vi "Byte Buffer.Clear.vi"(8 "error in (no error)":errorcluster, 11 "Byte Buffer in":refnum<class "Byte Buffer.lvclass">) -> (0 "error out":errorcluster, 3 "Byte Buffer out":refnum<class "Byte Buffer.lvclass">)   [LabVIEW 2016, in "VeriStand Data.lvlib" / "Byte Buffer.lvclass"]
doc: "Sets all bytes in the provided <B>buffer</B> to zero."
uses:
  Byte Buffer.lvclass
  Byte Buffer.lvclass/Byte Buffer.ctl
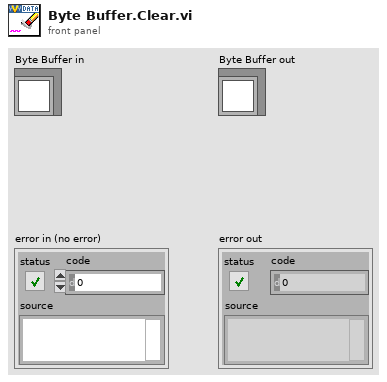
[diagram p1: front panel]
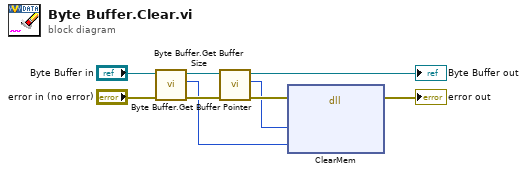
[diagram p0: block diagram]
diagram:
  n1 = call "Byte Buffer.Get Buffer Size.vi"("error in (no error)"="error in (no error)", "Byte Buffer in"="Byte Buffer in") -> ("error out"=w7:errorcluster, "buffer size"=w4:u64, "Byte Buffer out"=w2:refnum<class "Byte Buffer.lvclass">)  [unwired: 7 in]
  n2 = call "Byte Buffer.Get Buffer Pointer.vi"("error in (no error)"=w7, "Byte Buffer in"=w2) -> ("error out"=w6:errorcluster, "buffer pointer"=w5:u64, "Byte Buffer out"=→"Byte Buffer out":refnum<class "Byte Buffer.lvclass">)  [unwired: 7 in]
  n3 = dll-call lib="LabVIEW" fn="ClearMem"(error in=w6, "ptr"=w5, "size"=w4) -> (error out=→"error out":errorcluster)  [unwired: 5 in, 1 out]
